vi "Globals SS.vi"() -> ()   [LabVIEW 2016]
panel:
  in  "D L2 index":i32=7
  in  "C L2 index":i32=5
  in  "B L2 index":i32=3
  in  "A L2 Index":i32=1
  in  "D L1 index":i32=6
  in  "C L1 index":i32=4
  in  "B L1 index":i32=2
  in  "A L1 Index":i32
  in  "Max Len of Cyc":i32=32
  in  "Max Length of Display Data":i32=10000
  in  "Label Com Array":string[][](array[string])=[["M1", "100"], ["M3", "3"], ["M5", "5"], ["M7", "7"], ["M9", "9"], ["M11", "11"], ["M13", "13"], ["M15", "15"], ["M17", "17"], ["M19", "19"], ["M2", "2"], ["M4", "4"], ["M6", "6"], ["M8", "8"], ["M10", "10"], ["M12", "12"], ["M14", "14"], ["M16", "16"], ["M18", "18"], ["M20", "20"], ["N6", "21"], ["N7", "22"], ["N8", "23"], ["N9", "24"], ["N10", "25"], ["N11", "26"], ["N12", "27"], ["N13", "28"]]
  in  "Max Temp Alarm Limit":dbl=350.0
  in  "Fault Color":u32(colorbox)=16711680
  in  "Sub /R/N":string=" :: "
  in  "Save Data Array Length(56*11+1)":i32=617
  in  "Record Length for Sample Data":i32=11
  in  "Path: Data Backup":path=path "\\\\192.168.1.12\\share/Test Data/HCC"
  in  "Aisle Labels":string[](array[string])=["Aisle1", "Aisle2", "Aisle3"]
  in  "History Header Data":string[](array[string])=["Completion Time", "Cum Time On", "Imax(L1)", "Imax(L2)", "Temp(max)"]
  in  "Sample Header Data":string[](array[string])=["Time", "Cycle Count", "Cum Time On", "ASCII", "Status"]
  in  "UnConfigured":u32(colorbox)=7171459
  in  "Err Color":u32(colorbox)
  in  "Paused Color":u32(colorbox)=1985280
  in  "Unknown Status Color":u32(colorbox)
  in  "Running Color":u32(colorbox)=6618880
  in  "Not Started Color":u32(colorbox)=16776960
  in  "Stopped Color":u32(colorbox)=16776960
  in  "No Com Color":u32(colorbox)
  in  "No Com Status Message":string="No Com"
  in  "Path: Save File":path=path "C:/data"
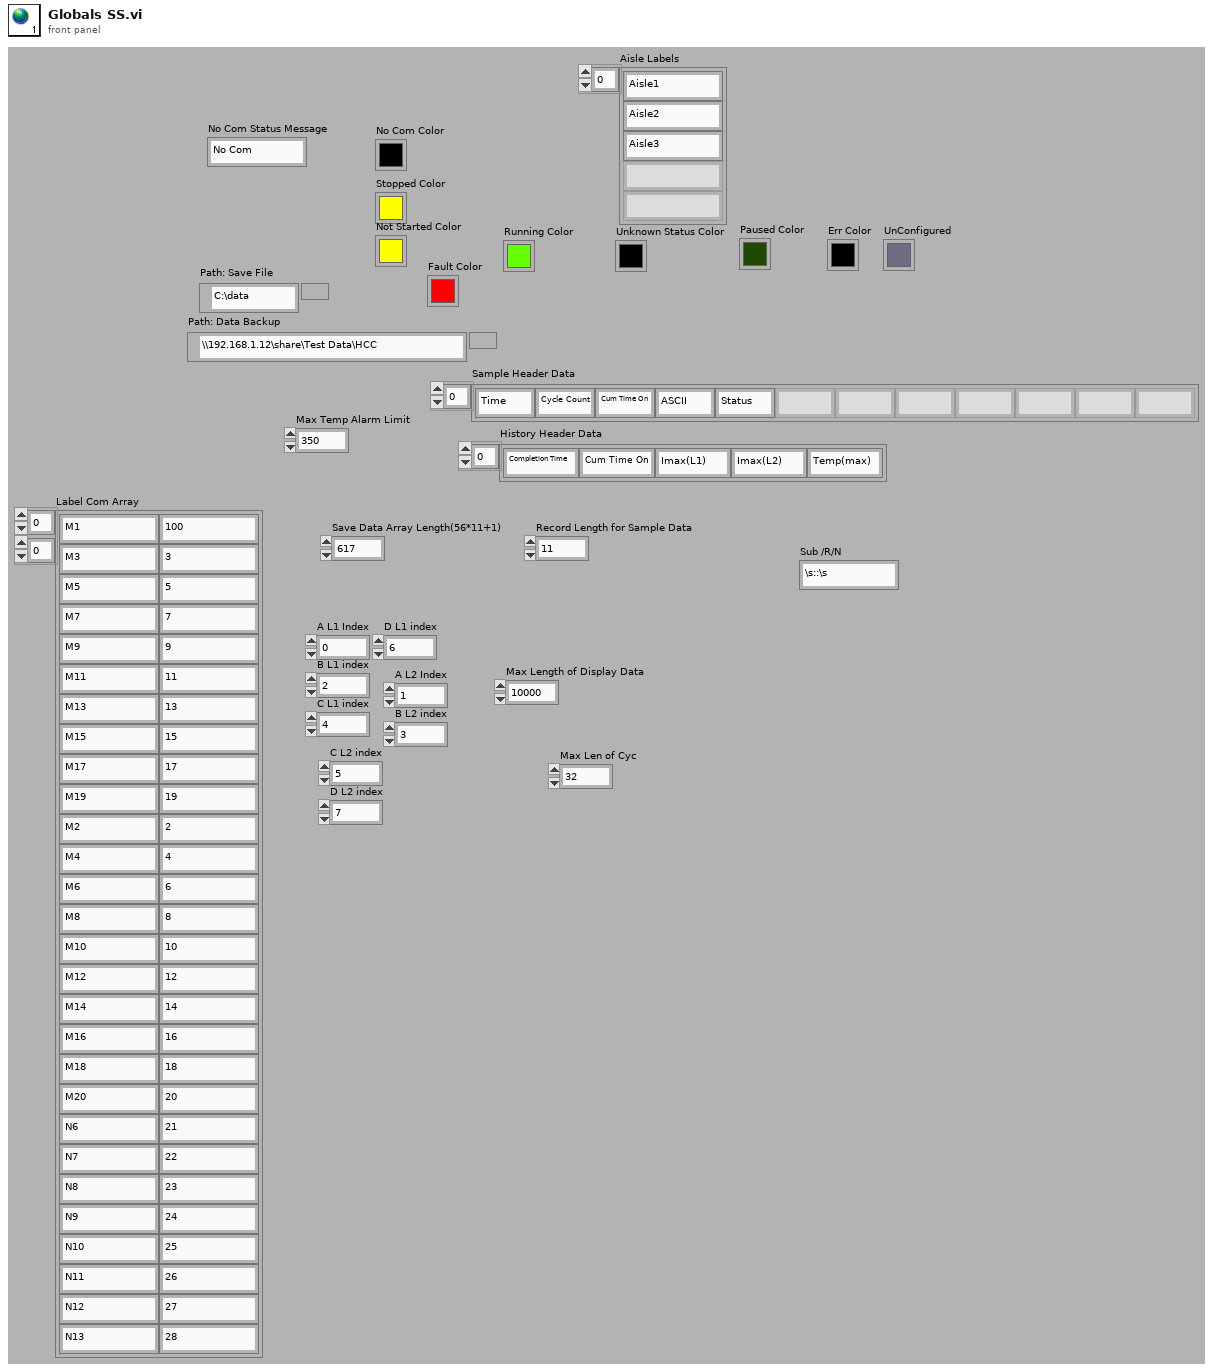
[diagram p1: front panel]
diagram:
